vi "Steam Out S&THx.vi"() -> ()   [LabVIEW 2017]
panel:
  out "Steam Out":dbl
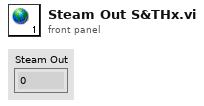
[diagram p1: front panel]
diagram:
